vi "Stop Core.vi"(10 "final error code":i32, 11 "Screw in":refnum<class "Screw.lvclass">) -> (3 "Screw out":refnum<class "Screw.lvclass">)   [LabVIEW 2018, in "Feeder Actor.lvlib" / "Screw.lvclass"]
doc: "(<B>Filename</B>: Actor Framework.lvlib:Actor.lvclass:Stop Core.vi)\n\nDefines what the actor does before it stops. Use the <B>final error code</B> input to determine whether the actor shut down in response to an error.\n\nBy default, this method passes the Stop message along to all auto-stop nested actors. A descendant class may override this method to define additional behavior, such as shutting down any processes the actor initiated in its override of the Actor Core method."
uses:
  Screw.lvclass
  Screw.lvclass/Screw.ctl
  <vilib>/MGI/Panel Manager/Panel Actor/Panel Actor/Panel Actor.lvclass
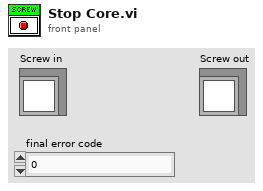
[diagram p1: front panel]
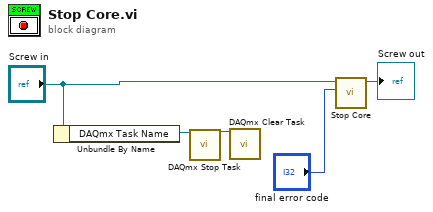
[diagram p0: block diagram]
diagram:
  n1 = Unbundle By Name("Screw in") -> ("DAQmx Task Name"=w2:refnum<k21>)
  n2 = call <vilib>:"DAQmx Stop Task.vi"("task/channels in"=w2) -> ("task out"=w3:refnum<k21>)  [unwired: 13 in, 1 out]
  n3 = call <vilib>:"DAQmx Clear Task.vi"("task in"=w3) -> ()  [unwired: 14 in, 1 out]
  n4 = call-parent "Stop Core.vi"("final error code"="final error code", "Monitored Actor in"="Screw in") -> ("Monitored Actor out"=→"Screw out":refnum<class "Screw.lvclass">)  [unwired: 9 in]
